vi "Main.vi"(11 "Module Admin":refnum<class "Delacor_lib_QMH_Module Admin.lvclass">) -> ()   [LabVIEW 2020, in "User Interfase.lvlib"]
doc: "This template is based off of the Queued Message Handler design pattern and the Queued Message Handler project template that ships with LabVIEW.\n\nThe main difference is that the queue is private to this module and communication between modules is performed via Broadcast and Request events.\n\nRequest events are wrapped in public API methods and are handled in the Event Handling Loop (EHL) of this VI. Any module can register for Broadcast events sent by this module. The EHL generates messages based on user interface actions.\n\nThe Message Handling Loop (MHL) processes messages generated by the EHL, or by other messages. The messages are string values, so new messages can be added easily to the Message Cases case structure in the MHL. Each message cluster can also provide an optional value for Message Data, which is a variant that can be converted to whatever message-specific data is required.\n_____\nBased on Delacor QMH Project Template 6.0.0.89."
uses:
  User Interfase.lvlib
  <vilib>/Delacor/Delacor QMH/Libraries/Module Admin_class/Delacor_lib_QMH_Module Admin.lvclass
  Module Data--cluster.ctl
  Stop Argument--cluster.ctl
  <vilib>/Delacor/Delacor QMH/Libraries/Message Queue_class/Delacor_lib_QMH_Message Queue.lvclass/Delacor_lib_QMH_Message Queue.ctl
  <vilib>/Delacor/Delacor QMH/Libraries/Module Admin_class/Delacor_lib_QMH_Module Admin.lvclass/Delacor_lib_QMH_Module Admin.ctl
  <vilib>/Delacor/Delacor QMH/Libraries/Message Queue_class/Delacor_lib_QMH_Enqueue Message (Single).vi
  <vilib>/Delacor/Delacor QMH/Libraries/Module Admin_class/Delacor_lib_QMH_Get External Launch.vi
  <vilib>/Utility/error.llb/Error Cluster From Error Code.vi
  <vilib>/ErrorRing/Error Ring.xnode
  <vilib>/Delacor/Delacor QMH/Libraries/Message Queue_class/Delacor_lib_QMH_Message Queue.lvclass
panel:
  out "ANALOGICO":dbl[](graph)
  out "Status":string
  out "Array":bool[](array[boolean])
  out "DIGITAL":dbl[](graph)
  out "error out":errorcluster
  in  "Play Button 2":bool
  in  "Play Button":bool
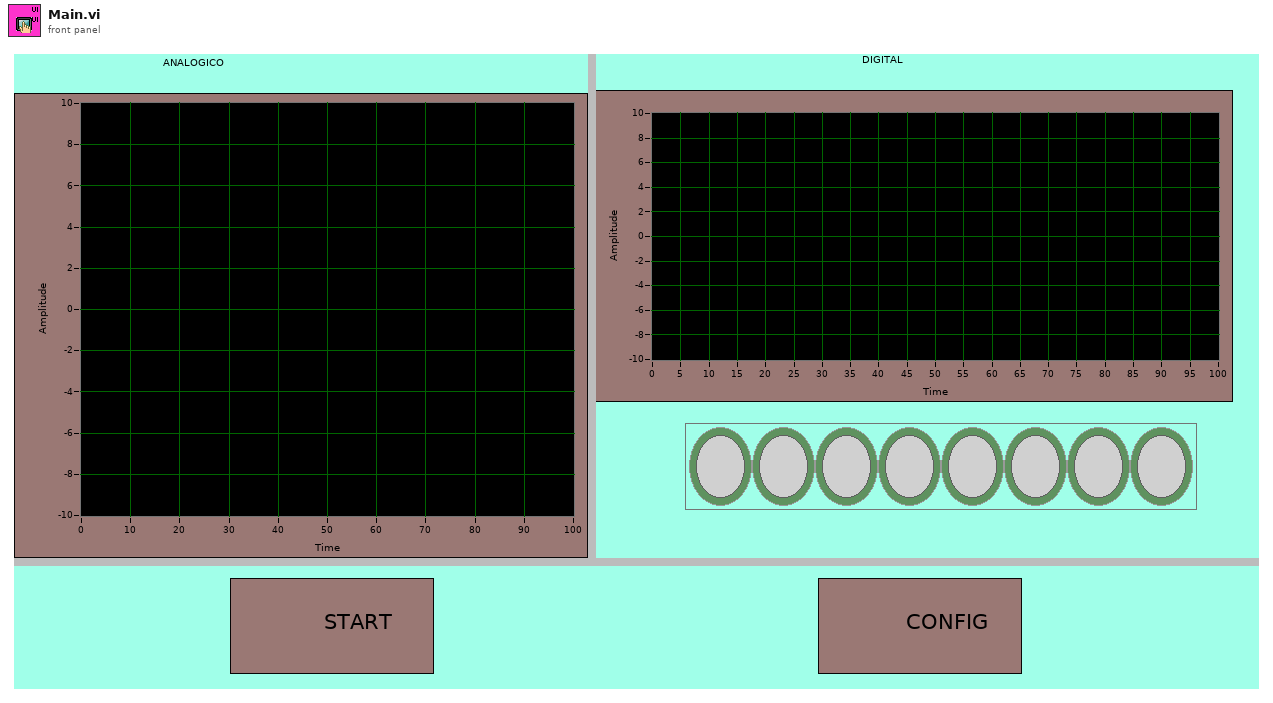
[diagram p1: front panel]
types:
  T1 = typedef "User Interfase.lvlib/Request Events--cluster.ctl" = cluster{"Stop Module":refnum<user-event>, "Show Panel":refnum<user-event>, "Hide Panel":refnum<user-event>, "Get Module Execution Status":refnum<user-event>, "Show Diagram":refnum<user-event>}
  T2 = typedef "User Interfase.lvlib/Module Data--cluster.ctl" = cluster{"Status":string}
  T3 = enum32{"invalid lock state", "Not Locked", "Locked (No Password)", "Password-protected"}
  T4 = typedef "User Interfase.lvlib/Stop Argument--cluster.ctl" = cluster{"Origin":string, "Exit via Stop Module Req?":bool, "Wait for Module to stop?":bool}
  T5 = enum32{"Invalid", "Standard", "Closed", "Hidden", "Minimized", "Maximized"}
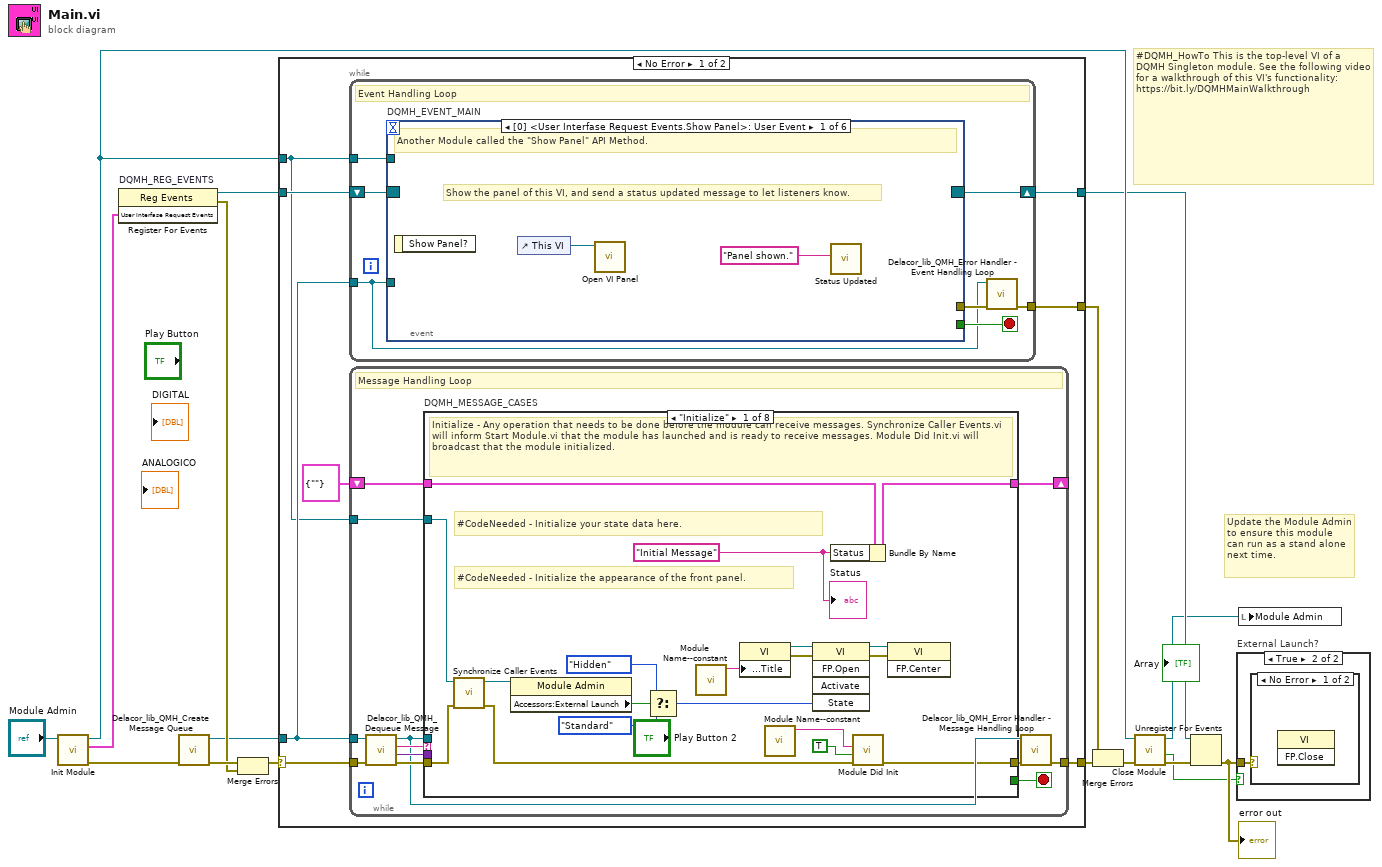
[diagram p0: block diagram]
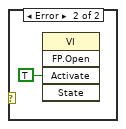
[diagram p3: hidden frame]
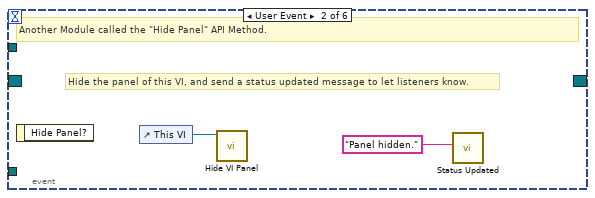
[diagram p4: hidden frame]
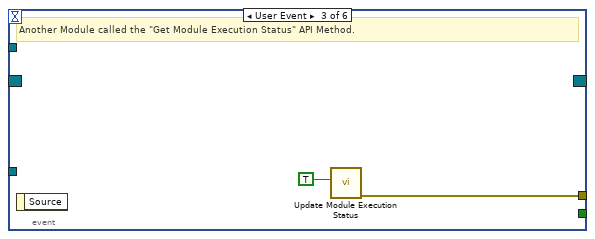
[diagram p5: hidden frame]
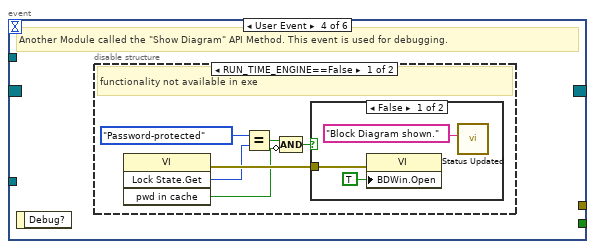
[diagram p6: hidden frame]
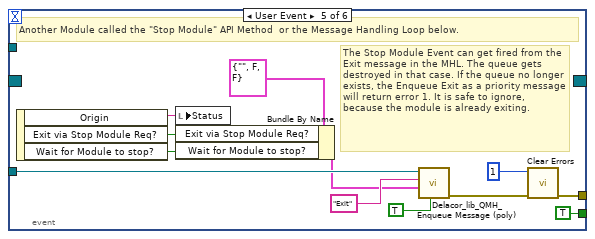
[diagram p9: hidden frame]
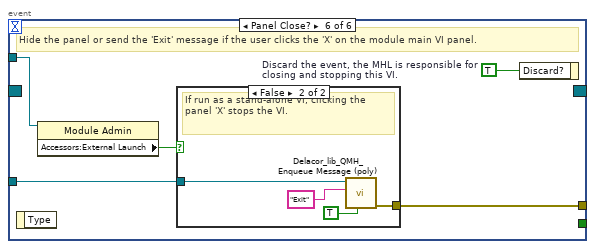
[diagram p10: hidden frame]
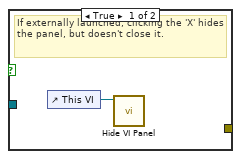
[diagram p11: hidden frame]
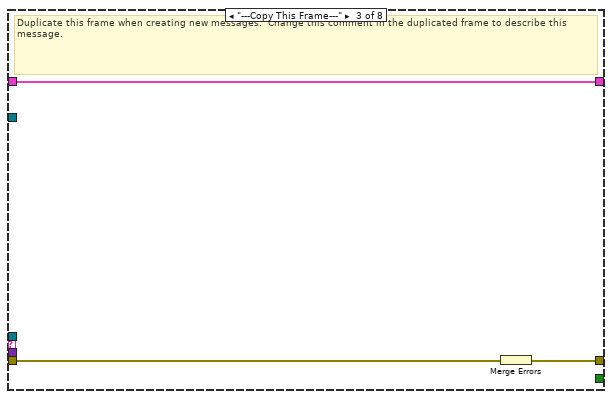
[diagram p13: hidden frame]
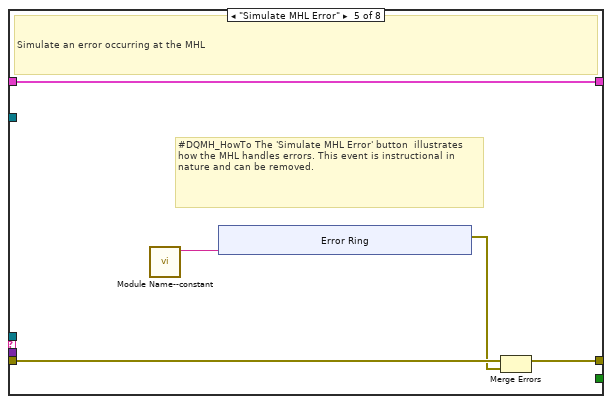
[diagram p15: hidden frame]
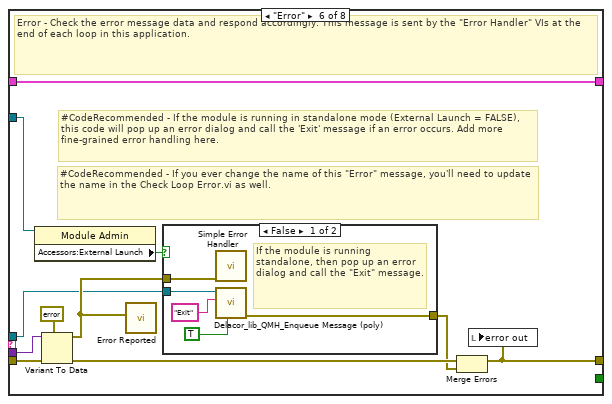
[diagram p16: hidden frame]
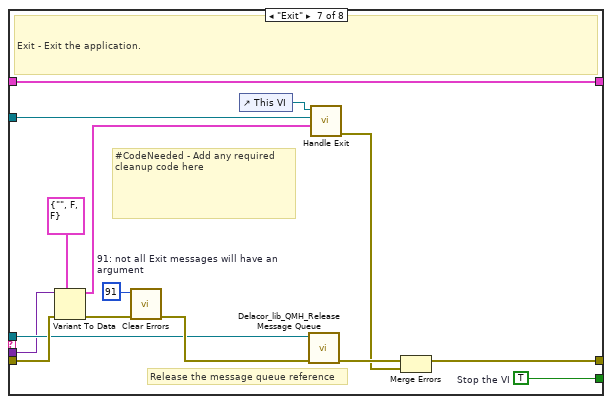
[diagram p18: hidden frame]
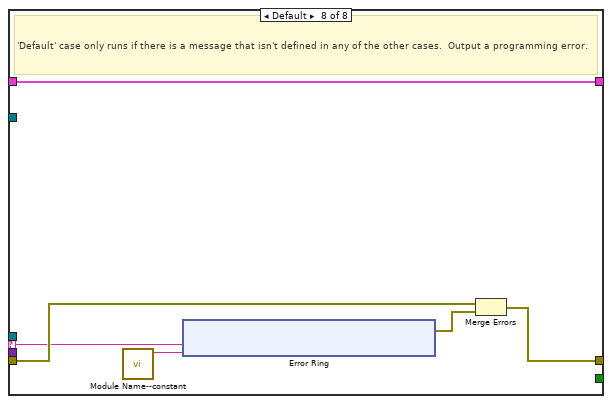
[diagram p19: hidden frame]
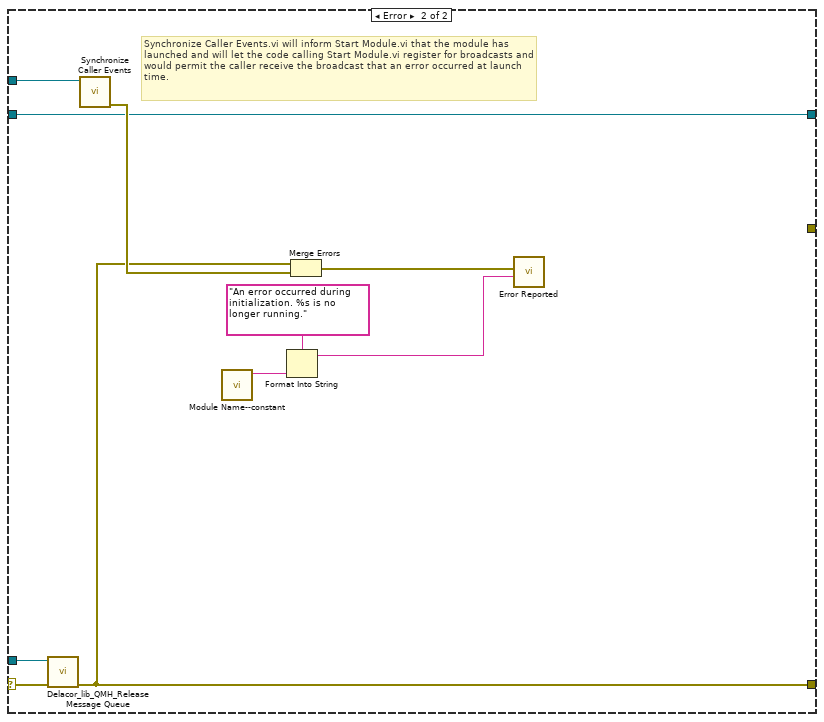
[diagram p20: hidden frame]
diagram:
  # "#DQMH_HowTo This is the top-level VI of a DQMH Singleton module. See the following video for a walkthrough of this VI's functionality: https://bit.ly/DQMHMainWalkthrough"
  # "Update the Module Admin to ensure this module can run as a stand alone next time."
  n1 = call "Init Module.vi"("Singleton Module Admin in"="Module Admin") -> ("error out"=w16:errorcluster, "User Interfase Request Events"=w5:T1, "Singleton Module Admin out"=w8:refnum<class "Delacor_lib_QMH_Module Admin.lvclass">)  [unwired: 8 in]
  n2 = register-events "DQMH_REG_EVENTS"(w5) -> (reference out=w6:refnum<event-registration>, error out=w9:errorcluster)  [unwired: 2 in]
  n3 = call <vilib>:"Delacor_lib_QMH_Create Message Queue.vi"("error in"=w16) -> ("error out"=w11:errorcluster, "Message Queue"=w4:refnum<class "Delacor_lib_QMH_Message Queue.lvclass">)  [unwired: 9 in]
  n4 = Merge Errors(w11, w9) -> (w10:errorcluster)
  n5 = case shown="No Error" w10 {
    selector: w10 -> [w23 w167]
    tunnel: [w25 w166] -> w17
    tunnel: [w22 w172] -> w7
    tunnel: w6 -> [w20 w172]
    tunnel: w4 -> [w19 w165]
    tunnel: [w24 _] -> w14
    tunnel: w8 -> [w18 w168]
    frame No Error {
      n6 = while {
        tunnel: w19 -> [w26]
        shift-right: [w29] -> w22
        shift-left: w20 -> [w30]
        tunnel: [w31] -> w24
        tunnel: w18 -> [w27]
        stop <- w28 stop-if-true
        # "Event Handling Loop"
        n7 = event "DQMH_EVENT_MAIN" shown="[0] <User Interfase Request Events.Show Panel>: User Event" {
          selector: w30 -> [_ _ _ _ _ _]
          dyn-events: [_ _ _ _ _ _] -> w29
          timeout: _ -> [_ _ _ _ _ _]
          tunnel: [_ _ _ _ TRUE ("Discard?") _] -> w28
          tunnel: w26 -> [_ _ _ _ w55 w62]
          tunnel: [_ _ w38 _ w58 w64] -> w32
          tunnel: w27 -> [_ _ _ _ _ w61]
          event User Event {
            # "Show the panel of this VI, and send a status updated message to let listeners know."
            # "Another Module called the \"Show Panel\" API Method."
            n8 = event-data() -> ()  [unwired: 1 in, 1 out]
            n9 = control-ref of="This VI"() -> (w34:refnum<vi>)
            n10 = call "Open VI Panel.vi"("VI"=w34) -> ()  [unwired: 10 in, 1 out]
            n11 = call "Status Updated.vi"("Status"="Panel shown." ("format string")) -> ()  [unwired: 10 in, 1 out]
          }
          event User Event {
            # "Hide the panel of this VI, and send a status updated message to let listeners know."
            # "Another Module called the \"Hide Panel\" API Method."
            n12 = event-data() -> ()  [unwired: 1 in, 1 out]
            n13 = control-ref of="This VI"() -> (w36:refnum<vi>)
            n14 = call "Hide VI Panel.vi"("VI"=w36) -> ()  [unwired: 10 in, 1 out]
            n15 = call "Status Updated.vi"("Status"="Panel hidden." ("format string")) -> ()  [unwired: 10 in, 1 out]
          }
          event User Event {
            # "Another Module called the \"Get Module Execution Status\" API Method."
            n16 = event-data() -> ()  [unwired: 1 in, 1 out]
            n17 = call "Update Module Execution Status.vi"("Running?"=TRUE) -> ("error out"=w38:errorcluster)  [unwired: 10 in]
          }
          event User Event {
            # "Another Module called the \"Show Diagram\" API Method. This event is used for debugging."
            n18 = event-data() -> ()  [unwired: 1 in, 1 out]
            n19 = disable-structure shown="RUN_TIME_ENGINE==False" {
              frame condition #0 (active) {
                # "functionality not available in exe"
                n20 = invoke class="VI" method="Lock State.Get"() -> (error out=w44:errorcluster, "Get Lock State"=w43:T3, "pwd in cache"=w40:bool)  [unwired: 4 in, 1 out]
                n21 = Equal?(x=T3."Password-protected", y=w43) -> (x = y?=w41:bool)
                n22 = Compound Arithmetic op=AND(w41, invert w40) -> (w39:bool)
                n23 = case shown="False" w39 {
                  tunnel: w44 -> [w47 _]
                  frame False {
                    n24 = property class="VI"(error in=w47, "BDWin.Open"=TRUE ("Block Diagram Window:Open")) -> ()  [unwired: 1 in, 2 out]
                    n25 = call "Status Updated.vi"("Status"="Block Diagram shown." ("format string")) -> ()  [unwired: 10 in, 1 out]
                  }
                  frame True {
                    # "Password-protected VI, and the password is not in the cache. Do not show the diagram."
                  }
                }
              }
              frame condition #1 {
              }
            }
          }
          event User Event {
            # "The Stop Module Event can get fired from the Exit message in the MHL. The queue gets destroyed in that case. If the queue no longer exists, the Enqueue Exit as a priority message will return error 1. It is safe to ignore, because the module is already exiting."
            # "Another Module called the \"Stop Module\" API Method  or the Message Handling Loop below."
            n26 = event-data() -> ("Origin"=w54:string, "Exit via Stop Module Req?"=w50:bool, "Wait for Module to stop?"=w49:bool)  [unwired: 1 in]
            n27 = local write "Status"(w54) -> ()
            n28 = Bundle By Name(cluster=T4 {"Origin"="", "Exit via Stop Module Req?"=FALSE, "Wait for Module to stop?"=FALSE} ("Stop Argument"), "Exit via Stop Module Req?"=w50, "Wait for Module to stop?"=w49) -> (w48:T4)
            n29 = call-poly <vilib>:"Delacor_lib_QMH_Enqueue Message (poly).vi"("Priority Message? (F)"=TRUE, "Message Data"=w48, "Message"="Exit", "Message Queue in"=w55) -> ("error out"=w59:errorcluster)  [unwired: 6 in, 1 out]
            n30 = call <vilib>:"Clear Errors.vi"("error in (no error)"=w59, "specific error code to clear (0: all)"=1) -> ("error out"=w58:errorcluster)  [unwired: 4 in, 1 out]
          }
          event Panel Close? {
            w63 = TRUE  # Discard the event, the MHL is responsible for closing and stopping this VI.
            # "Hide the panel or send the 'Exit' message if the user clicks the 'X' on the module main VI panel."
            n31 = event-data() -> ()  [unwired: 1 in, 1 out]
            n32 = property class="Module Admin"(reference=w61) -> ("Accessors:External Launch"=w60:bool)  [unwired: 1 in, 2 out]
            n33 = case shown="False" w60 {
              tunnel: w62 -> [_ w68]
              tunnel: [_ w69] -> w64
              frame True {
                # "If externally launched, clicking the 'X' hides the panel, but doesn't close it."
                n34 = control-ref of="This VI"() -> (w65:refnum<vi>)
                n35 = call "Hide VI Panel.vi"("VI"=w65) -> ()  [unwired: 10 in, 1 out]
              }
              frame False {
                # "If run as a stand-alone VI, clicking the panel 'X' stops the VI."
                n36 = call-poly <vilib>:"Delacor_lib_QMH_Enqueue Message (poly).vi"("Priority Message? (F)"=TRUE, "Message"="Exit", "Message Queue in"=w68) -> ("error out"=w69:errorcluster)  [unwired: 7 in, 1 out]
              }
            }
            n37 = event-data("Discard?"=w63) -> ()  [unwired: 1 in, 1 out]
          }
        }
        n38 = call-dynamic "Delacor_lib_QMH_Error Handler - Event Handling Loop.vi"("error in"=w32, "Message Queue in"=w26) -> ("dup error in"=w31:errorcluster)  [unwired: 8 in, 1 out]
      }
      n39 = while {
        tunnel: w19 -> [w72]
        shift-right: [w76] -> _
        shift-left: T2 {"Status"=""} ("Data Cluster") -> [w77]
        tunnel: w23 -> [w80]
        tunnel: [w78] -> w25
        tunnel: w18 -> [w70]
        stop <- w75 stop-if-true
        # "Message Handling Loop"
        n40 = call-dynamic "Delacor_lib_QMH_Dequeue Message.vi"("error in"=w80, "Message Queue in"=w72) -> ("error out"=w79:errorcluster, "Message Data"=w73:variant, "Message"=w74:string, "Message Queue out"=w71:refnum<class "Delacor_lib_QMH_Message Queue.lvclass">)  [unwired: 6 in]
        n41 = case "DQMH_MESSAGE_CASES" shown="\"Initialize\"" w74 {
          selector: w74 -> [_ _ _ _ _ _ _ w152]
          tunnel: w71 -> [_ _ _ _ _ w122 w144 _]
          tunnel: w79 -> [w98 w102 w105 w107 w112 w129 w150 w154]
          tunnel: [w96 w102 w104 w107 w111 w125 w147 w155] -> w81
          tunnel: w77 -> [w87 w101 w103 w106 w109 w124 w143 w153]
          tunnel: [w86 w101 w103 w106 w109 w124 w143 w153] -> w76
          tunnel: [_ _ _ _ _ _ w142 _] -> w75
          tunnel: w73 -> [_ _ _ _ _ w123 w141 _]
          tunnel: w70 -> [w88 _ _ _ _ w121 w136 _]
          frame "Initialize" {
            w82 = "Initial Message" ("Initial Message")
            # "#CodeNeeded - Initialize the appearance of the front panel."
            # "#CodeNeeded - Initialize your state data here."
            # "Initialize - Any operation that needs to be done before the module can receive messages. Synchronize Caller Events.vi will inform Start Module.vi that the module has launched and is ready to receive messages. Module Did Init.vi will broadcast that the module initialized."
            n42 = call "Synchronize Caller Events.vi"("error in (no error)"=w98, "Singleton Module Admin in"=w88) -> ("error out"=w97:errorcluster, "Singleton Module Admin out"=w83:refnum<class "Delacor_lib_QMH_Module Admin.lvclass">)  [unwired: 8 in]
            n43 = property class="Module Admin"(reference=w83) -> ("Accessors:External Launch"=w92:bool)  [unwired: 1 in, 2 out]
            n44 = Select(t=T5."Hidden" ("State"), s=w92, f=T5."Standard" ("State")) -> (s? t:f=w89:T5)
            n45 = call "Module Name--constant.vi"() -> ("Module Name"=w95:string)  [unwired: 11 in]
            n46 = property class="VI"("Front Panel.Title"=w95) -> (reference out=w94:refnum<vi>, error out=w100:errorcluster)  [unwired: 2 in]
            n47 = call "Module Name--constant.vi"() -> ("Module Name"=w84:string)  [unwired: 11 in]
            n48 = invoke class="VI" method="FP.Open"(reference=w94, error in=w100, "State"=w89) -> (reference out=w93:refnum<vi>, error out=w99:errorcluster)  [unwired: 2 in, 3 out]
            n49 = Bundle By Name(cluster=w87, "Status"=w82) -> (w86:T2)
            n50 = call "Module Did Init.vi"("error in (no error)"=w97, "Initialized?"=TRUE, "Origin"=w84) -> ("error out"=w96:errorcluster)  [unwired: 8 in]
            n51 = invoke class="VI" method="FP.Center"(reference=w93, error in=w99) -> ()  [unwired: 1 in, 3 out]
            "Status" <- w82
          }
          frame "---Module Specific---" {
            # "Separator -- The following cases handle messages specific to this Module."
          }
          frame "---Copy This Frame---" {
            # "Duplicate this frame when creating new messages.  Change this comment in the duplicated frame to describe this message."
            n52 = Merge Errors(w105) -> (w104:errorcluster)
          }
          frame "---Exit and Error Handling---" {
            # "Separator - The following cases handle errors and exit messages."
          }
          frame "Simulate MHL Error" {
            # "#DQMH_HowTo The 'Simulate MHL Error' button  illustrates how the MHL handles errors. This event is instructional in nature and can be removed."
            # "Simulate an error occurring at the MHL"
            n53 = call "Module Name--constant.vi"() -> ("Module Name"=w108:string)  [unwired: 11 in]
            n54 = xnode "Error Ring"("parameter 0"=w108) -> ("error out"=w110:errorcluster)
            n55 = Merge Errors(w112, w110) -> (w111:errorcluster)
          }
          frame "Error" {
            # "#CodeRecommended - If you ever change the name of this \"Error\" message, you'll need to update the name in the Check Loop Error.vi as well."
            # "#CodeRecommended - If the module is running in standalone mode (External Launch = FALSE), this code will pop up an error dialog and call the 'Exit' message if an error occurs. Add more fine-grained error handling here."
            # "Error - Check the error message data and respond accordingly. This message is sent by the \"Error Handler\" VIs at the end of each loop in this application."
            n56 = property class="Module Admin"(reference=w121) -> ("Accessors:External Launch"=w120:bool)  [unwired: 1 in, 2 out]
            n57 = Variant To Data(error in=w129, type=errorcluster {"status"=FALSE, "code"=0, "source"=""} ("error constant"), Variant=w123) -> (data=w130:errorcluster, error out=w127:errorcluster)
            n58 = call "Error Reported.vi"("Error"=w130) -> ()  [unwired: 10 in, 1 out]
            n59 = case shown="False" w120 {
              tunnel: [w135 _] -> w126
              tunnel: w122 -> [w133 _]
              tunnel: w130 -> [w134 _]
              frame False {
                # "If the module is running standalone, then pop up an error dialog and call the \"Exit\" message."
                n60 = call <vilib>:"Simple Error Handler.vi"("error in (no error)"=w134) -> ()  [unwired: 4 in, 5 out]
                n61 = call-poly <vilib>:"Delacor_lib_QMH_Enqueue Message (poly).vi"("Priority Message? (F)"=TRUE, "Message"="Exit", "Message Queue in"=w133) -> ("error out"=w135:errorcluster)  [unwired: 7 in, 1 out]
              }
              frame True {
                # "If the module was launched externally, calling the Error Reported broadcast VI is the only action performed by the \"Error\" message. The module's caller can then process the error appropriately."
              }
            }
            n62 = Merge Errors(w127, w126) -> (w125:errorcluster)
            n63 = local write "error out"(w125) -> ()
          }
          frame "Exit" {
            w140 = 91  # 91: not all Exit messages will have an argument
            w142 = TRUE  # Stop the VI
            # "Release the message queue reference"
            # "#CodeNeeded - Add any required cleanup code here"
            # "Exit - Exit the application."
            n64 = Variant To Data(error in=w150, type=T4 {"Origin"="", "Exit via Stop Module Req?"=FALSE, "Wait for Module to stop?"=FALSE} ("Stop Argument"), Variant=w141) -> (data=w138:T4, error out=w146:errorcluster)
            n65 = call <vilib>:"Clear Errors.vi"("error in (no error)"=w146, "specific error code to clear (0: all)"=w140) -> ("error out"=w149:errorcluster)  [unwired: 4 in, 1 out]
            n66 = control-ref of="This VI"() -> (w137:refnum<vi>)
            n67 = call-dynamic "Delacor_lib_QMH_Release Message Queue.vi"("error in"=w149, "Message Queue"=w144) -> ("error out"=w148:errorcluster)  [unwired: 9 in]
            n68 = call "Handle Exit.vi"("Stop Argument"=w138, "Admin in"=w136, "VI reference"=w137) -> ("error out"=w145:errorcluster)  [unwired: 7 in, 1 out]
            n69 = Merge Errors(w148, w145) -> (w147:errorcluster)
          }
          frame Default {
            # "'Default' case only runs if there is a message that isn't defined in any of the other cases.  Output a programming error."
            n70 = call "Module Name--constant.vi"() -> ("Module Name"=w151:string)  [unwired: 11 in]
            n71 = xnode "Error Ring"("parameter 0"=w152, "parameter 1"=w151) -> ("error out"=w156:errorcluster)
            n72 = Merge Errors(w154, w156) -> (w155:errorcluster)
          }
        }
        n73 = call-dynamic "Delacor_lib_QMH_Error Handler - Message Handling Loop.vi"("error in"=w81, "Message Queue in"=w71) -> ("dup error in"=w78:errorcluster)  [unwired: 8 in, 1 out]
      }
    }
    frame Error {
      # "Synchronize Caller Events.vi will inform Start Module.vi that the module has launched and will let the code calling Start Module.vi register for broadcasts and would permit the caller receive the broadcast that an error occurred at launch time."
      n74 = call-dynamic "Delacor_lib_QMH_Release Message Queue.vi"("error in"=w167, "Message Queue"=w165) -> ("error out"=w166:errorcluster)  [unwired: 9 in]
      n75 = call "Synchronize Caller Events.vi"("Singleton Module Admin in"=w168) -> ("error out"=w173:errorcluster)  [unwired: 9 in, 1 out]
      n76 = call "Module Name--constant.vi"() -> ("Module Name"=w171:string)  [unwired: 11 in]
      n77 = Format Into String(format string="An error occurred during initialization. %s is no longer running.", w171) -> (resulting string=w169:string)  [unwired: 2 in, 1 out]
      n78 = Merge Errors(w166, w173) -> (w174:errorcluster)
      n79 = call "Error Reported.vi"("Additional Information"=w169, "Error"=w174) -> ()  [unwired: 9 in, 1 out]
    }
  }
  n80 = Merge Errors(w14, w17) -> (w13:errorcluster)
  n81 = call "Close Module.vi"("error in (no error)"=w13, "Module Admin in"=w8) -> ("error out"=w15:errorcluster, "External Launch"=w1:bool, "Module Admin out"=w2:refnum<class "Delacor_lib_QMH_Module Admin.lvclass">)  [unwired: 7 in]
  n82 = Unregister For Events(event registration refnum=w7, error in=w15) -> (error out=w12:errorcluster)
  "error out" <- w12
  n83 = case "External Launch?" shown="True" w1 {
    tunnel: w12 -> [_ w175]
    frame False {
    }
    frame True {
      n84 = case shown="No Error" w175 {
        frame No Error {
          n85 = invoke class="VI" method="FP.Close"() -> ()  [unwired: 3 in, 3 out]
        }
        frame Error {
          n86 = invoke class="VI" method="FP.Open"("Activate"=TRUE ("Activate?")) -> ()  [unwired: 4 in, 5 out]
        }
      }
    }
  }
  n87 = local write "Module Admin"(w2) -> ()
